vi "Init.vi"(8 "error in (no error)":errorcluster, 11 "Car in":refnum<class "Car.lvclass">) -> (0 "error out":errorcluster, 3 "Car out":refnum<class "Car.lvclass">)   [LabVIEW 2019, in "Car.lvclass"]
uses:
  Car.lvclass
  Vehicle/Vehicle.lvclass/Vehicle.ctl
  Vehicle/Vehicle.lvclass
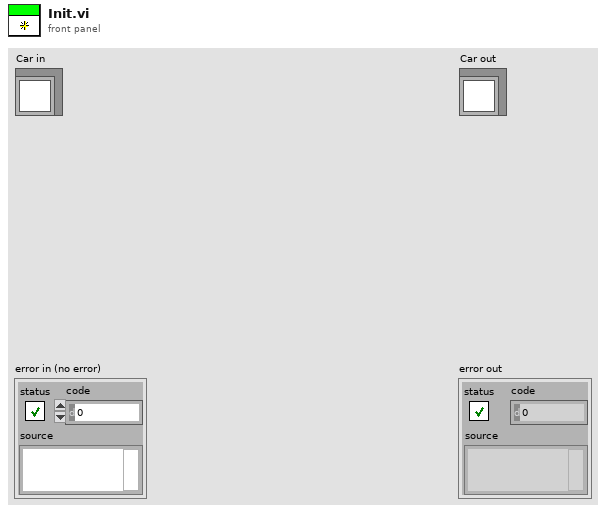
[diagram p1: front panel]
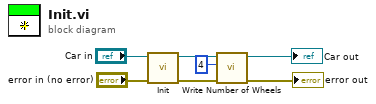
[diagram p0: block diagram]
diagram:
  n1 = call-parent "Init.vi"("error in (no error)"="error in (no error)", "Vehicle in"="Car in") -> ("error out"=w5:errorcluster, "Vehicle out"=w4:refnum<class "Car.lvclass">)  [unwired: 8 in]
  n2 = call "Write Number of Wheels .vi"("error in (no error)"=w5, "Number of Wheels"=4, "Vehicle in"=w4) -> ("error out"=→"error out":errorcluster, "Vehicle out"=→"Car out":refnum<class "Car.lvclass">)  [unwired: 7 in]
